vi "live view D04.vi"() -> ()   [LabVIEW 2019, in "D04.lvlib"]
uses:
  D04.lvlib
  <vilib>/userDefined/High Color/IMAQdx.ctl
  <vilib>/vision/Image Controls.llb/IMAQ Image.ctl
  <vilib>/measure/mamon.llb/Trigger Detection for 1 Channel.vi
  <vilib>/measure/NI_MAPro.lvlib
  Calibration Lib.lvlib
  database.lvlib
  <vilib>/vision/driver/NI_Vision_Acquisition_Software.lvlib
panel:
  out "Error out":errorcluster
  in  "Save Button":bool
  in  "Calib IMQ Num":u16(ring) items=["First IMQ", "Second IMQ", "Third IMQ"]
  in  "Verify Calibration1 D04":bool caption="capture grab"
  in  "snapshot":bool
  out "error prj03":errorcluster
  in  "Verify Calibration D04":bool caption="capture grab"
  in  "Close":bool
  in  "Method 2 save D04":bool caption="capture grab"
  in  "Method 1 Save D04":bool caption="Saving txt"
  out "Average Result":string="Average Result"
  out ">18  A":dbl(slide)=1.0 caption=">16 mm" scale=0.0..100.0
  out "16-18  A":dbl(slide)=1.0 caption="14-16 mm" scale=0.0..100.0
  out "14-16  A":dbl(slide)=1.0 caption="12.7-14 mm" scale=0.0..100.0
  out "12.5-14 A":dbl(slide)=1.0 caption="11-12.7 mm" scale=0.0..100.0
  out "10-12.5  A":dbl(slide)=1.0 caption="9.5-11 mm" scale=0.0..100.0 scale format="%#_4f"
  out "8-10  A":dbl(slide)=1.0 caption="8-9.5 mm" scale=0.0..100.0
  out "6.3-8  A":dbl(slide)=1.0 caption="6.3-8 mm" scale=0.0..100.0
  out "<6.3  A":dbl(slide)=1.0 caption="<6.3 mm" scale=0.0..100.0
  out "Live Result":string="Live Result"
  out ">18  L":dbl(slide)=1.0 caption=">16 mm" scale=0.0..100.0
  out "Live View":T1(plugin-control) caption="Disc 26"
  out "16-18  L":dbl(slide)=1.0 caption="14-16 mm" scale=0.0..100.0
  out "14-16  L":dbl(slide)=1.0 caption="12.7-14 mm" scale=0.0..100.0
  out "12.5-14 L":dbl(slide)=1.0 caption="11-12.7 mm" scale=0.0..100.0
  out "10-12.5  L":dbl(slide)=1.0 caption="9.5-11 mm" scale=0.0..100.0 scale format="%#_4f"
  out "8-10  L":dbl(slide)=1.0 caption="8-9.5 mm" scale=0.0..100.0
  out "6.3-8  L":dbl(slide)=1.0 caption="6.3-8 mm" scale=0.0..100.0
  out "<6.3  L":dbl(slide)=1.0 caption="<6.3 mm" scale=0.0..100.0
  out "disc name":string="Live Info Disc 04"
  out "dsgs":string="DSGS"
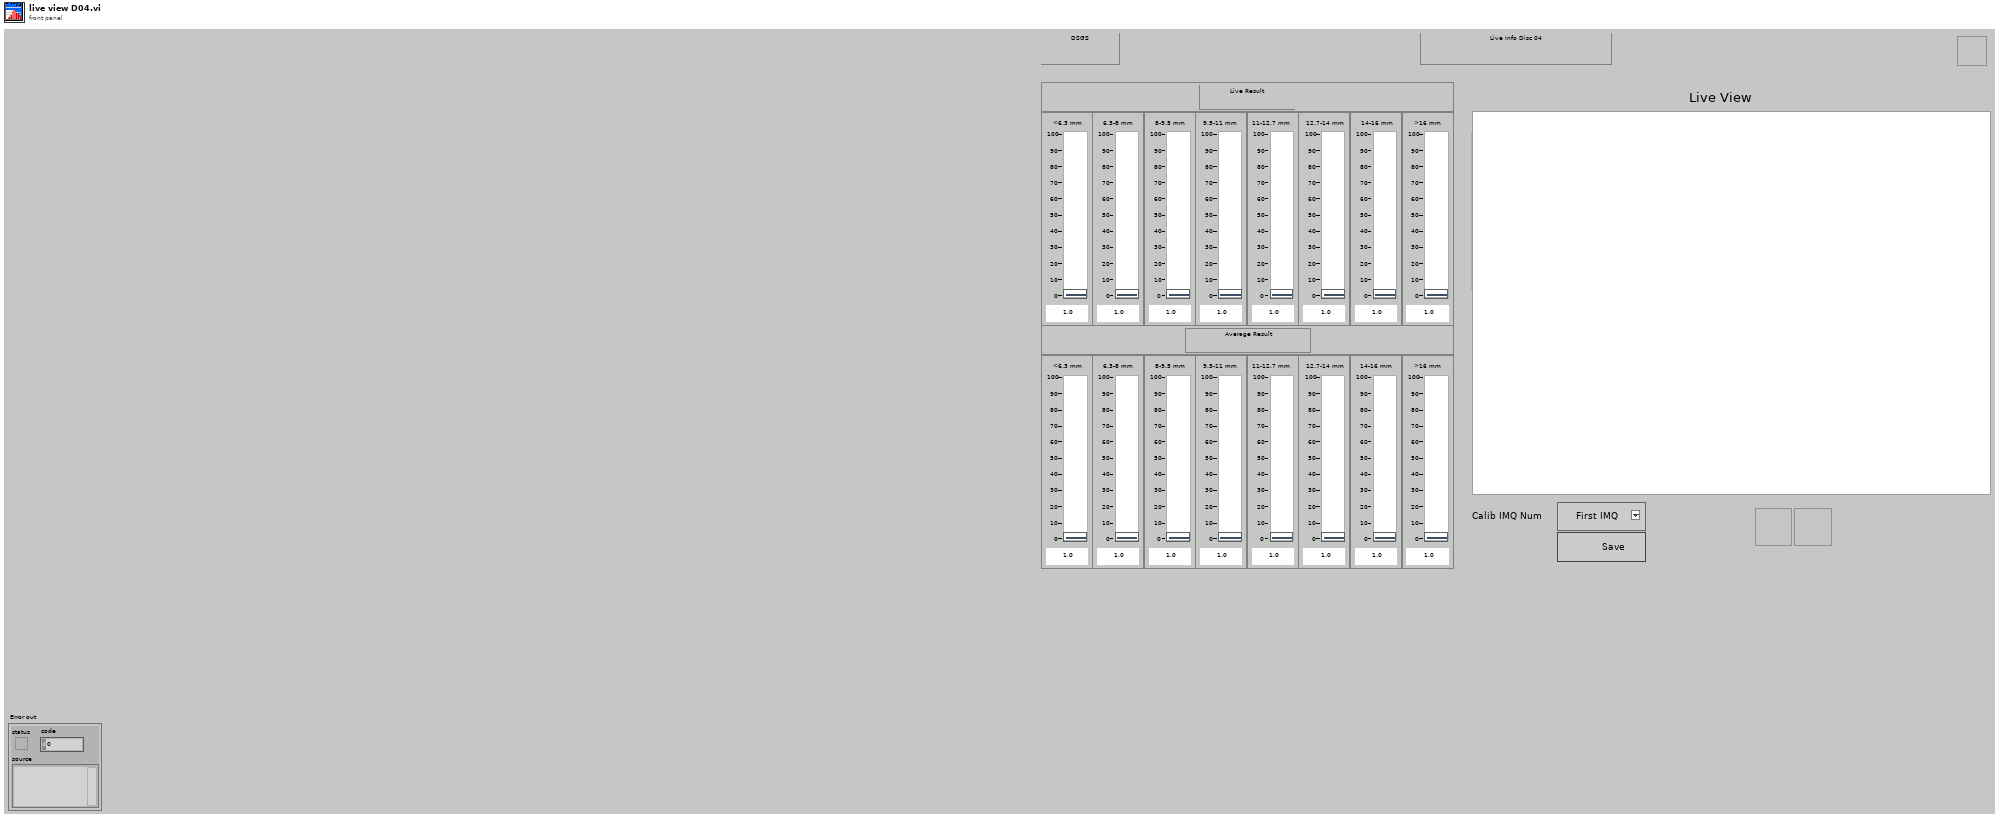
[diagram p1: front panel]
types:
  T1 = typedef "IMAQ Image.ctl" = refnum<image>
  T2 = typedef "IMAQdx.ctl" = refnum<k21>
  T3 = enum8{"Enabled", "Disabled", "Disabled and Grayed Out"}
  T4 = cluster{"date/time string":string, "date/time string":string, string, "Value":dbl, "Value":dbl, "Value":dbl, "Value":dbl, "Value":dbl, "Value":dbl, "Value":dbl, "Value":dbl}
  T5 = cluster{"date/time string":string, "date/time string":string, i32, "spreadsheet string":string, "spreadsheet string":string}
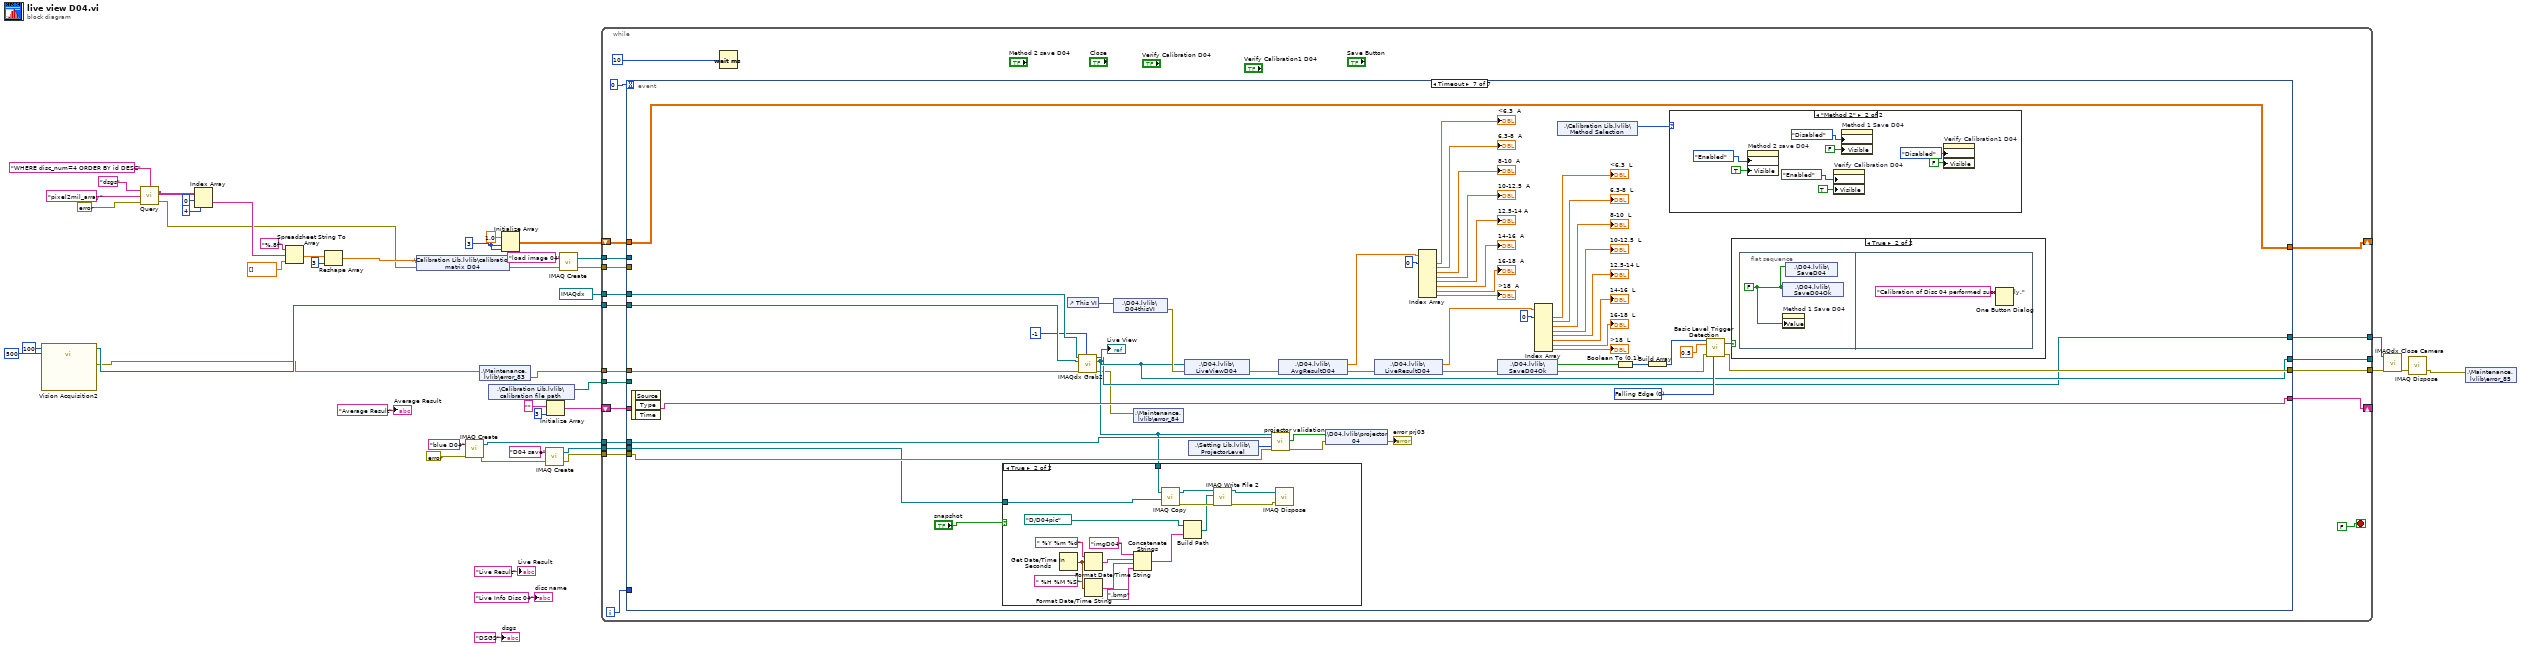
[diagram p0: block diagram]
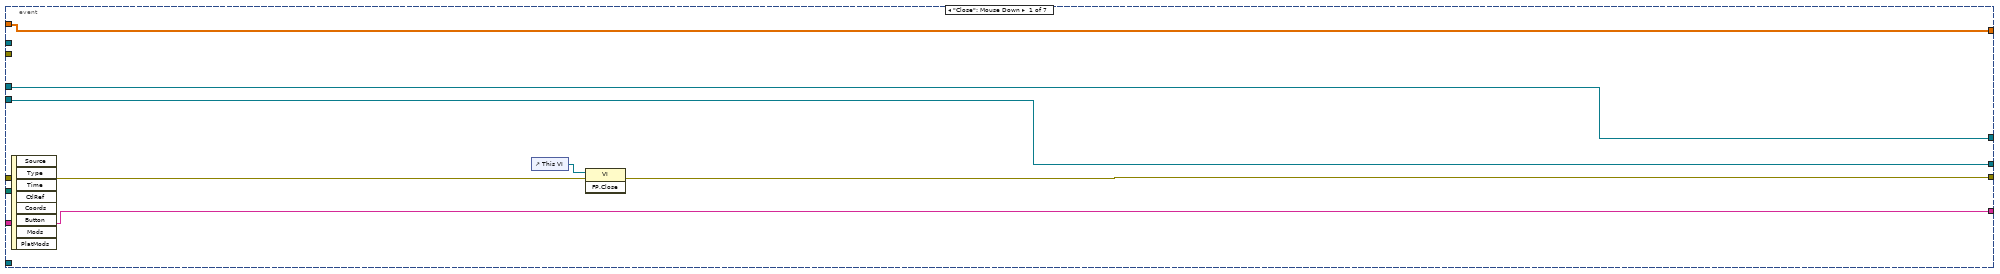
[diagram p2: hidden frame]
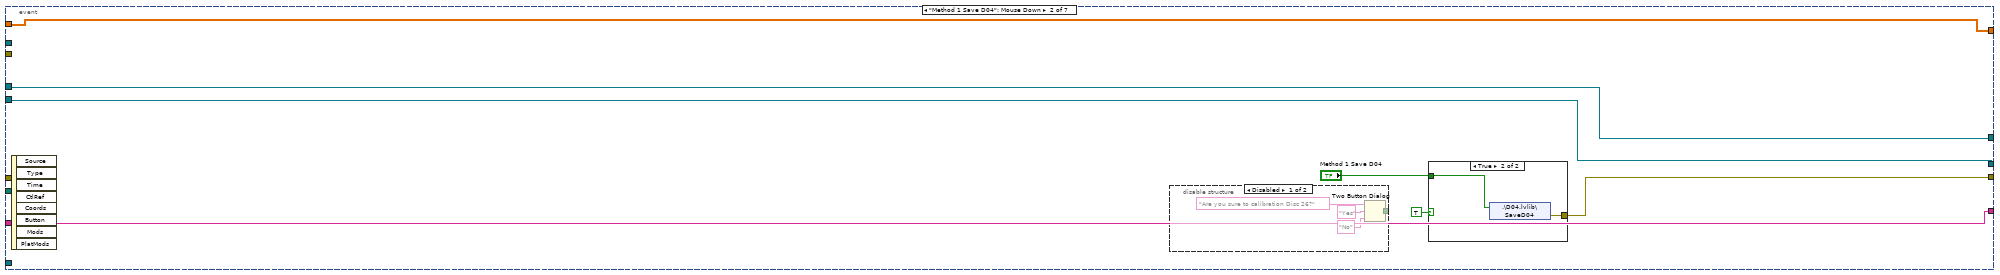
[diagram p3: hidden frame]
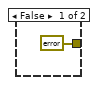
[diagram p5: hidden frame]
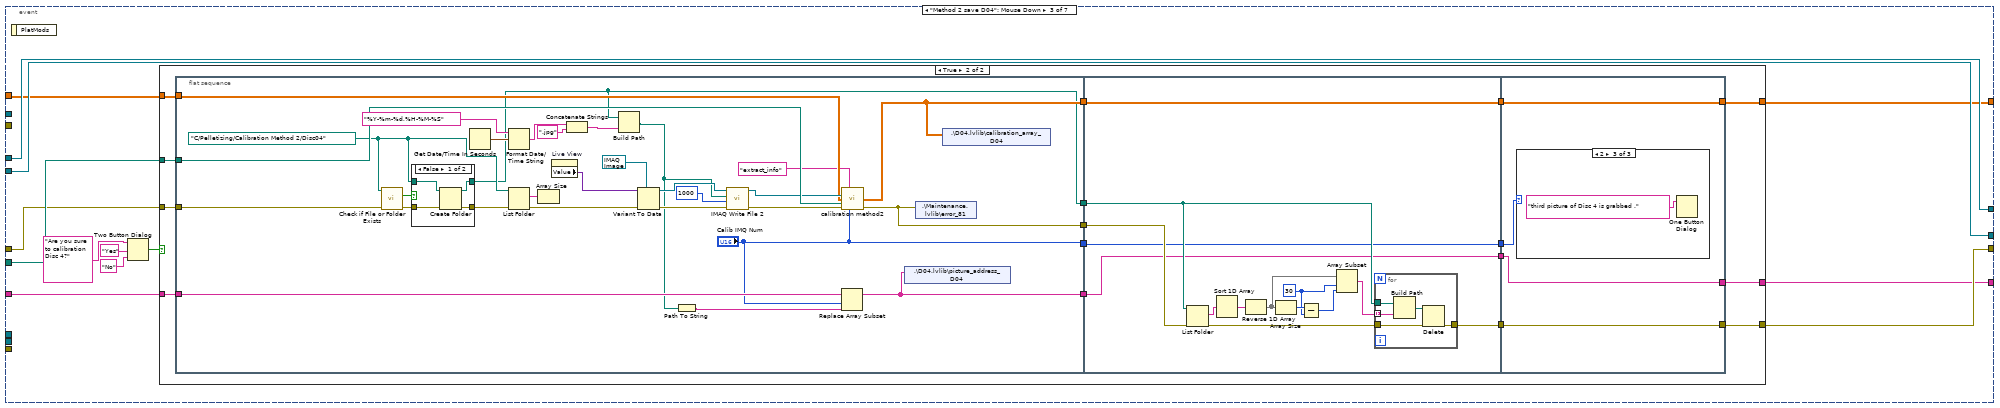
[diagram p6: hidden frame]
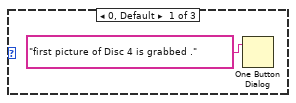
[diagram p9: hidden frame]
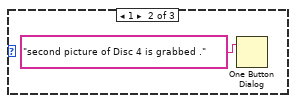
[diagram p10: hidden frame]
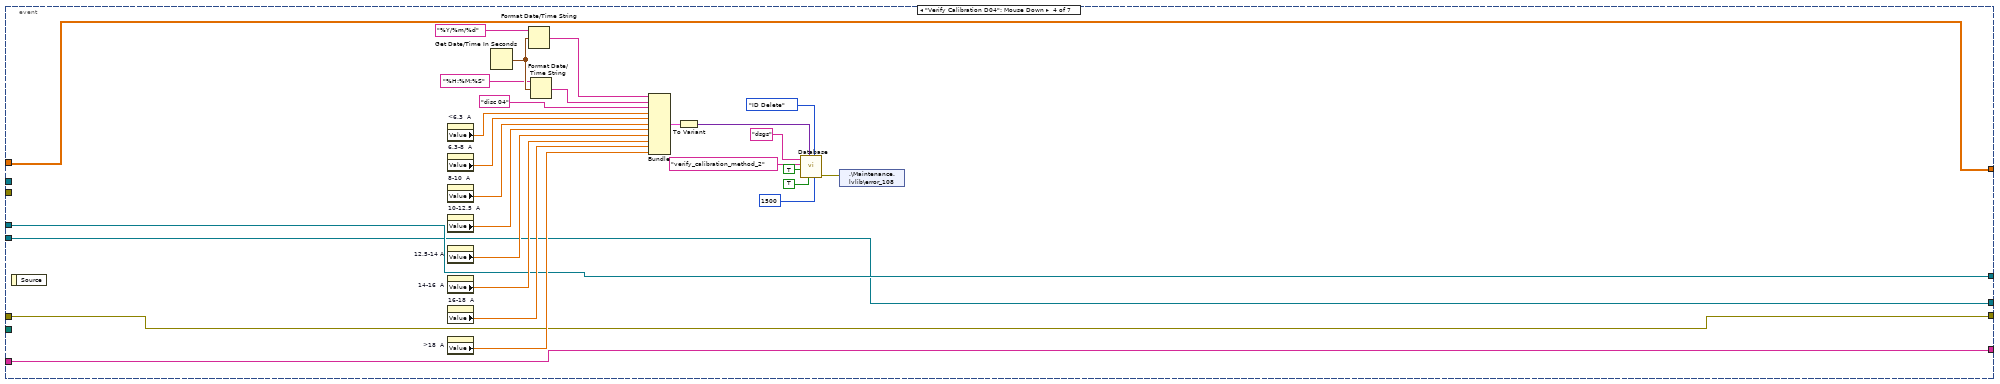
[diagram p11: hidden frame]
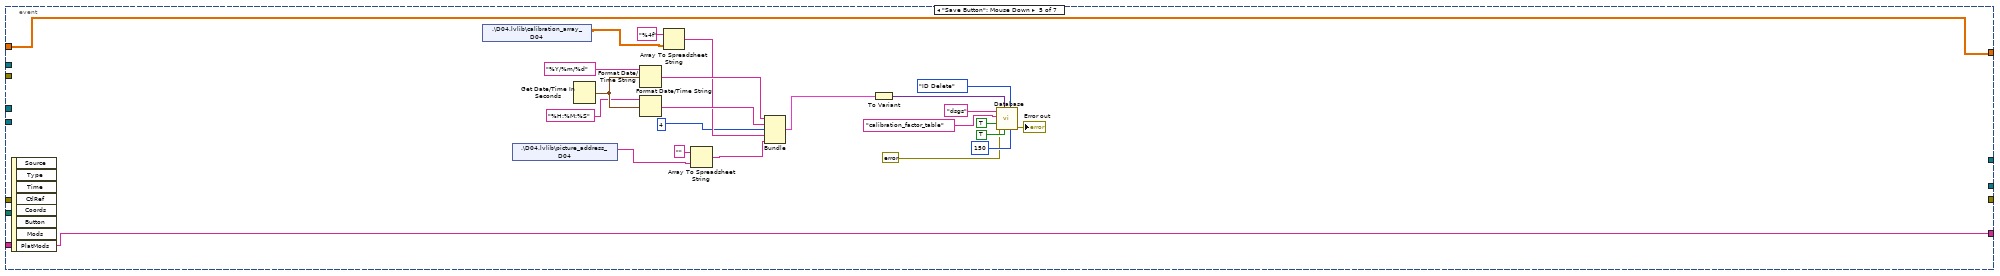
[diagram p12: hidden frame]
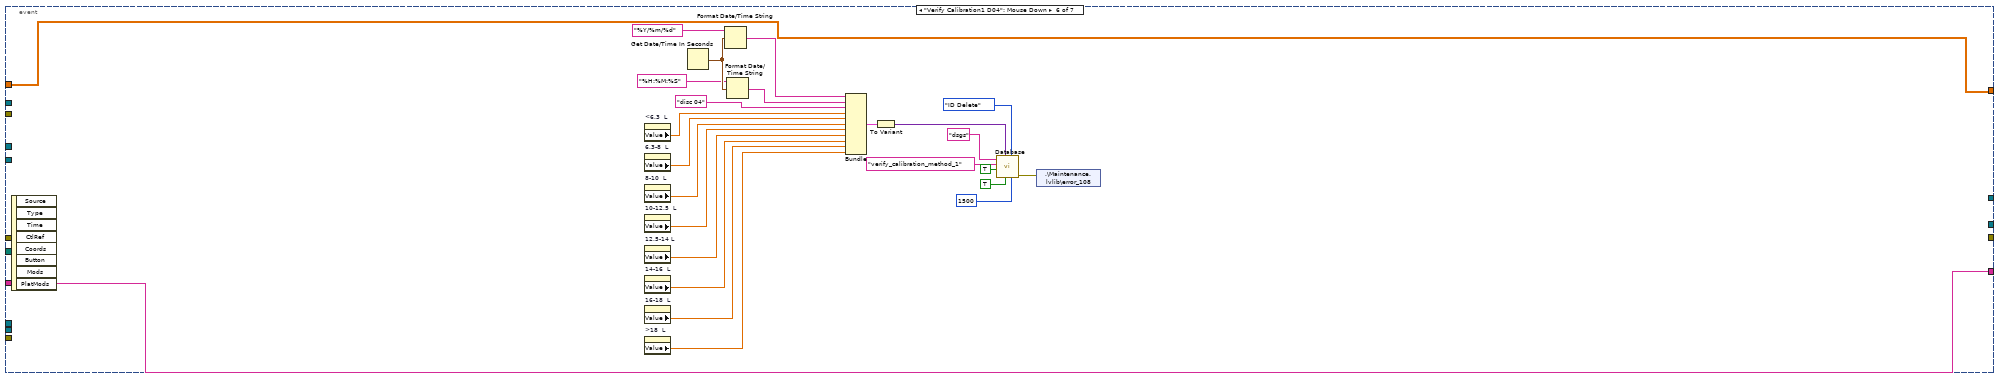
[diagram p13: hidden frame]
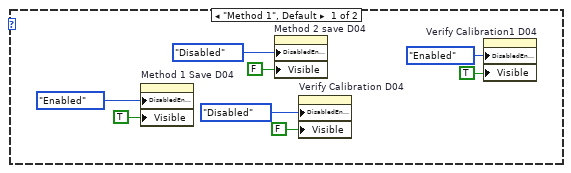
[diagram p15: hidden frame]
diagram:
  w15 = 3 ("dimension size")
  n1 = call "Vision Acquisition2"("Gain (Raw)"=i64 100, "Exposure Time (Raw)"=i64 500) -> ("Image Out"=w4:T1, "error out"=w3:errorcluster)  [unwired: 23 in, 1 out]
  n2 = call "Query.vi"("Condition"="WHERE disc_num=4 ORDER BY id DESC", "Error in"=errorcluster {"status"=FALSE, "code"=0, "source"=""}, "Table Name"="pixel2mil_array", "Connection Name"="dsgs") -> ("Error out"=w7:errorcluster, "data"=w10:string[][])
  n3 = Index Array(array=w10, index (row)=0, index (col)=4 ("disabled index (col)")) -> (element=w8:string)
  n4 = Spreadsheet String To Array(format string="%.8f", spreadsheet string=w8, array type (2D Dbl)=sgl[] []) -> (array=w28:sgl[])  [unwired: 1 in]
  n5 = Reshape Array(w28, 3 ("dimension size")) -> (w25:sgl[])
  n6 = shared-variable ".\\Calibration Lib.lvlib\\calibration matrix D04"(w25, error in=w7) -> (error out=w24:errorcluster)
  n7 = call "IMAQ Create"("Image Name"="blue D04", "error in (no error)"=errorcluster {"status"=FALSE, "code"=0, "source"=""}) -> ("New Image"=w22:T1, "error out"=w20:errorcluster)  [unwired: 3 in]
  n8 = shared-variable ".\\Maintenance.lvlib\\error_83"(w3) -> (error out=w37:errorcluster)  [unwired: 1 in]
  n9 = shared-variable ".\\Calibration Lib.lvlib\\calibration file path"() -> (w38:path)  [unwired: 1 in, 1 out]
  n10 = Initialize Array(1.0 ("element"), w15, w15) -> (w14:dbl[][])
  n11 = call "IMAQ Create"("Image Name"="D04 save", "error in (no error)"=w20) -> ("New Image"=w17:T1, "error out"=w19:errorcluster)  [unwired: 3 in]
  n12 = Initialize Array("", 3 ("dimension size")) -> (w11:string[])
  n13 = call "IMAQ Create"("Image Name"="load image 04", "error in (no error)"=w24) -> ("New Image"=w34:T1, "error out"=w35:errorcluster)  [unwired: 3 in]
  n14 = while {
    tunnel: w38 -> [w64]
    tunnel: w37 -> [w63]
    tunnel: w4 -> [w61]
    tunnel: [w60] -> w42
    tunnel: [w59] -> _
    tunnel: T2 "cam3" ("Session In") -> [w58]
    tunnel: [w57] -> w39
    tunnel: w35 -> [w56]
    tunnel: w34 -> [w55]
    tunnel: w22 -> [w54]
    tunnel: w19 -> [w53]
    tunnel: w17 -> [w52]
    shift-right: [w49] -> _
    shift-left: w14 -> [w50]
    shift-right: [w47] -> _
    shift-left: w11 -> [w48]
    i -> [w51]
    stop <- FALSE stop-if-true
    n15 = event shown="[6] Timeout" {
      selector: _ -> [_ _ _ _ _ _ _]
      dyn-events: _ -> [_ _ _ _ _ _ _]
      timeout: 0 -> [_ _ _ _ _ _ _]
      tunnel: w64 -> [_ _ w100 _ _ _ _]
      tunnel: [w72 w80 w96 w188 _ _ w277] -> w60
      tunnel: w63 -> [w71 _ w99 w188 _ _ w262]
      tunnel: w61 -> [w70 w79 w98 w186 _ _ w261]
      tunnel: [w70 w79 w98 w186 _ _ w265] -> w59
      tunnel: w58 -> [w69 w78 w97 w187 _ _ w264]
      tunnel: [w69 w78 w97 w187 _ _ w263] -> w57
      tunnel: w56 -> [_ _ _ _ _ _ _]
      tunnel: w55 -> [_ _ _ _ _ _ _]
      tunnel: w54 -> [_ _ _ _ _ _ w275]
      tunnel: w53 -> [_ _ _ _ _ _ w271]
      tunnel: w52 -> [_ _ _ _ _ _ w268]
      tunnel: w51 -> [_ _ _ _ _ _ _]
      tunnel: w50 -> [w68 w75 w91 w183 w212 w235 w267]
      tunnel: [w68 w75 w90 w183 w212 w235 w267] -> w49
      tunnel: w48 -> [w67 w74 w89 w182 w211 w234 w266]
      tunnel: [w67 w74 w88 w182 w211 w234 w266] -> w47
      event "Close": Mouse Down {
        n16 = event-data() -> ()  [unwired: 1 in, 8 out]
        n17 = control-ref of="This VI"() -> (w73:refnum<vi>)
        n18 = invoke class="VI" method="FP.Close"(reference=w73, error in=w71) -> (error out=w72:errorcluster)  [unwired: 1 in, 2 out]
      }
      event "Method 1 Save D04": Mouse Down {
        n19 = event-data() -> ()  [unwired: 1 in, 8 out]
        n20 = disable-structure shown="Disabled" {
          disable-tunnel: [w81 _] -> _
          frame Disabled {
            n21 = Two Button Dialog(message="Are you sure to calibration Disc 26?", 1:"No" ("F button name (\"Cancel\")"), 2:"Yes" ("T button name (\"OK\")")) -> (T button?=w81:bool)
          }
          frame Enabled {
          }
        }
        n22 = case shown="True" TRUE {
          tunnel: [errorcluster {"status"=FALSE, "code"=0, "source"=""} ("error IO") w87] -> w80
          tunnel: "Method 1 Save D04" -> [_ w86]
          frame False {
          }
          frame True {
            n23 = shared-variable ".\\D04.lvlib\\SaveD04"(w86) -> (error out=w87:errorcluster)  [unwired: 1 in]
          }
        }
      }
      event "Method 2 save D04": Mouse Down {
        n24 = event-data() -> ()  [unwired: 1 in, 1 out]
        n25 = Two Button Dialog(message="Are you sure to calibration Disc 4?", 1:"No" ("F button name (\"Cancel\")"), 2:"Yes" ("T button name (\"OK\")")) -> (T button?=w92:bool)
        n26 = case shown="True" w92 {
          tunnel: w100 -> [_ w118]
          tunnel: w99 -> [w103 w117]
          tunnel: [w103 w116] -> w96
          tunnel: w91 -> [w102 w114]
          tunnel: [w102 w111] -> w90
          tunnel: w89 -> [w101 w110]
          tunnel: [w101 w107] -> w88
          frame False {
          }
          frame True {
            n27 = flat-sequence {
              tunnel: w117 -> [w138]
              tunnel: w118 -> [w149]
              tunnel: [w123] -> w119
              tunnel: w114 -> [w131]
              tunnel: [w130] -> w112
              tunnel: w110 -> [w127]
              tunnel: [w126] -> w108
              tunnel: [w125] -> w106
              tunnel: ["Calib IMQ Num"] -> w104
              tunnel: [w160] -> w115
              tunnel: [w158] -> w113
              tunnel: [w157] -> w109
              tunnel: w106 -> [w161]
              tunnel: w108 -> [w157]
              tunnel: w112 -> [w158]
              tunnel: w119 -> [w162]
              tunnel: [w156] -> w105
              tunnel: w104 -> [w156]
              tunnel: [w178] -> w116
              tunnel: w115 -> [w178]
              tunnel: [w177] -> w111
              tunnel: w113 -> [w177]
              tunnel: [w176] -> w107
              tunnel: w109 -> [w176]
              tunnel: w105 -> [w175]
              frame #0 {
                w134 = path "C:/Pelletizing/Calibration Method 2/Disc04" ("path")
                n28 = call <vilib>:"Check if File or Folder Exists.vi"("error in (no error)"=w138, "path"=w134) -> ("error out"=w139:errorcluster, "file or folder exists?"=w140:bool)  [unwired: 7 in, 1 out]
                n29 = case shown="False" w140 {
                  tunnel: [w151 w155] -> w123
                  tunnel: w134 -> [w153 w155]
                  tunnel: w139 -> [w152 w154]
                  tunnel: [w150 w154] -> w136
                  frame False {
                    n30 = Create Folder(path (use dialog)=w153, error in=w152) -> (created path=w151:path, error out=w150:errorcluster)  [unwired: 1 in, 1 out]
                  }
                  frame True {
                  }
                }
                n31 = Get Date/Time In Seconds() -> (seconds since 1Jan1904=w144:timestamp)
                n32 = Format Date/Time String(time format string (%c)="%Y-%m-%d,%H-%M-%S", seconds (now)=w144) -> (date/time string=w142:string)  [unwired: 1 in]
                n33 = List Folder(path=w134, error in=w136) -> (filenames=w137:string[], error out=w135:errorcluster)  [unwired: 2 in, 2 out]
                n34 = Array Size(array=w137) -> ()  [unwired: 1 out]
                n35 = property on="Live View" class="ImageControl"() -> ("Value"=w148:variant)  [unwired: 2 in, 2 out]
                n36 = Concatenate Strings(w142, ".jpg" ("string")) -> (w124:string)
                n37 = Build Path(base path=w123, name or relative path=w124) -> (appended path=w121:path)
                n38 = Variant To Data(error in=w135, type=T1 refnum ("New Image"), Variant=w148) -> (data=w132:T1, error out=w145:errorcluster)
                n39 = Path To String(path=w121) -> (string=w122:string)
                n40 = call-poly "IMAQ Write File 2"("error in (no error)"=w145, "Image Quality"=u32 1000, "File Path"=w121, "Image"=w132) -> ("error out"=w129:errorcluster, "Image Out (duplicate)"=w133:T1)  [unwired: 6 in]
                n41 = Replace Array Subset(array=w127, new element=w122, index="Calib IMQ Num") -> (w126:string[])
                n42 = call "calibration method2.vi"("function name"="extract_info", "Image IN"=w133, "initialize matrix"=w131, "module path"=w149, "error in"=w129, "snap number"="Calib IMQ Num") -> ("calibration matrix"=w130:dbl[][], "error out"=w125:errorcluster)  [unwired: 8 in]
                n43 = shared-variable ".\\D04.lvlib\\picture_address_D04"(w126) -> ()  [unwired: 1 in, 1 out]
                n44 = shared-variable ".\\Maintenance.lvlib\\error_81"(w125) -> ()  [unwired: 1 in, 1 out]
                n45 = shared-variable ".\\D04.lvlib\\calibration_array_D04"(w130) -> ()  [unwired: 1 in, 1 out]
              }
              frame #1 {
                w163 = 30 ("index")
                n46 = List Folder(path=w162, error in=w161) -> (filenames=w169:string[], error out=w159:errorcluster)  [unwired: 2 in, 2 out]
                n47 = Sort 1D Array(array=w169) -> (sorted array=w168:string[])
                n48 = Reverse 1D Array(array=w168) -> (reversed array=w167:string[])
                n49 = Array Size(array=w167) -> (size(s)=w166:i32)
                n50 = Subtract(x=w166, y=w163) -> (x-y=w165:i32)
                n51 = Array Subset(array=w167, index=w163, length=w165) -> (w164:string[])
                n52 = for {
                  tunnel: w164 -> [w173] mode=indexing
                  tunnel: w162 -> [w174]
                  tunnel: [w171] -> w160
                  tunnel: w159 -> [w170]
                  n53 = Build Path(base path=w174, name or relative path=w173) -> (appended path=w172:path)
                  n54 = Delete(path (use dialog)=w172, error in=w170) -> (error out=w171:errorcluster)  [unwired: 3 in, 2 out]
                }
              }
              frame #2 {
                n55 = case shown="2" w175 {
                  frame 0, Default {
                    n56 = One Button Dialog(message="first picture of Disc 4 is grabbed .") -> ()  [unwired: 1 in, 1 out]
                  }
                  frame 1 {
                    n57 = One Button Dialog(message="second picture of Disc 4 is grabbed .") -> ()  [unwired: 1 in, 1 out]
                  }
                  frame 2 {
                    n58 = One Button Dialog(message="third picture of Disc 4 is grabbed .") -> ()  [unwired: 1 in, 1 out]
                  }
                }
              }
            }
          }
        }
      }
      event "Verify Calibration D04": Mouse Down {
        n59 = event-data() -> ()  [unwired: 1 in, 1 out]
        n60 = property on="<6.3  A" class="Slide (strict)"() -> ("Value"=w203:dbl)  [unwired: 2 in, 2 out]
        n61 = property on="6.3-8  A" class="Slide (strict)"() -> ("Value"=w202:dbl)  [unwired: 2 in, 2 out]
        n62 = property on="8-10  A" class="Slide (strict)"() -> ("Value"=w201:dbl)  [unwired: 2 in, 2 out]
        n63 = property on="10-12.5  A" class="Slide (strict)"() -> ("Value"=w200:dbl)  [unwired: 2 in, 2 out]
        n64 = property on="12.5-14 A" class="Slide (strict)"() -> ("Value"=w199:dbl)  [unwired: 2 in, 2 out]
        n65 = property on="14-16  A" class="Slide (strict)"() -> ("Value"=w198:dbl)  [unwired: 2 in, 2 out]
        n66 = property on="16-18  A" class="Slide (strict)"() -> ("Value"=w197:dbl)  [unwired: 2 in, 2 out]
        n67 = property on=">18  A" class="Slide (strict)"() -> ("Value"=w196:dbl)  [unwired: 2 in, 2 out]
        n68 = Get Date/Time In Seconds() -> (seconds since 1Jan1904=w208:timestamp)
        n69 = Format Date/Time String(time format string (%c)="%Y/%m/%d", seconds (now)=w208) -> (date/time string=w206:string)  [unwired: 1 in]
        n70 = Format Date/Time String(time format string (%c)="%H:%M:%S", seconds (now)=w208) -> (date/time string=w205:string)  [unwired: 1 in]
        n71 = Bundle("date/time string"=w206, "date/time string"=w205, "disc 04", "Value"=w203, "Value"=w202, "Value"=w201, "Value"=w200, "Value"=w199, "Value"=w198, "Value"=w197, "Value"=w196) -> (w195:T4)  [unwired: 1 in]
        n72 = To Variant(anything=w195) -> (Variant=w194:variant)
        n73 = call "Database.vi"("Maximum Row"=1500, "Enum"=enum16{"ID Delete", "Time Delete"}."ID Delete", "Delete row?"=TRUE, "Data"=w194, "Auto Increment ID?"=TRUE, "Table"="verify_calibration_method_2", "Connection"="dsgs") -> ("Error out"=w189:errorcluster)  [unwired: 4 in]
        n74 = shared-variable ".\\Maintenance.lvlib\\error_108"(w189) -> ()  [unwired: 1 in, 1 out]
      }
      event "Save Button": Mouse Down {
        n75 = event-data() -> ()  [unwired: 1 in, 8 out]
        n76 = shared-variable ".\\D04.lvlib\\calibration_array_D04"() -> (w213:dbl[][])  [unwired: 1 in, 1 out]
        n77 = shared-variable ".\\D04.lvlib\\picture_address_D04"() -> (w215:string[])  [unwired: 1 in, 1 out]
        n78 = Get Date/Time In Seconds() -> (seconds since 1Jan1904=w222:timestamp)
        n79 = Format Date/Time String(time format string (%c)="%Y/%m/%d", seconds (now)=w222) -> (date/time string=w223:string)  [unwired: 1 in]
        n80 = Format Date/Time String(time format string (%c)="%H:%M:%S", seconds (now)=w222) -> (date/time string=w221:string)  [unwired: 1 in]
        n81 = Array To Spreadsheet String(array=w213, 3:"%4f" ("format string")) -> (spreadsheet string=w217:string)  [unwired: 1 in]
        n82 = Array To Spreadsheet String(array=w215, 3:"" ("format string")) -> (spreadsheet string=w214:string)  [unwired: 1 in]
        n83 = Bundle("date/time string"=w223, "date/time string"=w221, 4, "spreadsheet string"=w217, "spreadsheet string"=w214) -> (w226:T5)  [unwired: 1 in]
        n84 = To Variant(anything=w226) -> (Variant=w233:variant)
        n85 = call "Database.vi"("Maximum Row"=150, "Enum"=enum16{"ID Delete", "Time Delete"}."ID Delete", "Delete row?"=TRUE, "Data"=w233, "Error in"=errorcluster {"status"=FALSE, "code"=0, "source"=""}, "Auto Increment ID?"=TRUE, "Table"="calibration_factor_table", "Connection"="dsgs") -> ("Error out"=→"Error out":errorcluster)  [unwired: 3 in]
      }
      event "Verify Calibration1 D04": Mouse Down {
        n86 = event-data() -> ()  [unwired: 1 in, 8 out]
        n87 = property on="<6.3  L" class="Slide (strict)"() -> ("Value"=w252:dbl)  [unwired: 2 in, 2 out]
        n88 = property on="6.3-8  L" class="Slide (strict)"() -> ("Value"=w251:dbl)  [unwired: 2 in, 2 out]
        n89 = property on="8-10  L" class="Slide (strict)"() -> ("Value"=w250:dbl)  [unwired: 2 in, 2 out]
        n90 = property on="10-12.5  L" class="Slide (strict)"() -> ("Value"=w249:dbl)  [unwired: 2 in, 2 out]
        n91 = property on="12.5-14 L" class="Slide (strict)"() -> ("Value"=w248:dbl)  [unwired: 2 in, 2 out]
        n92 = property on="14-16  L" class="Slide (strict)"() -> ("Value"=w247:dbl)  [unwired: 2 in, 2 out]
        n93 = property on="16-18  L" class="Slide (strict)"() -> ("Value"=w246:dbl)  [unwired: 2 in, 2 out]
        n94 = property on=">18  L" class="Slide (strict)"() -> ("Value"=w245:dbl)  [unwired: 2 in, 2 out]
        n95 = Get Date/Time In Seconds() -> (seconds since 1Jan1904=w257:timestamp)
        n96 = Format Date/Time String(time format string (%c)="%Y/%m/%d", seconds (now)=w257) -> (date/time string=w255:string)  [unwired: 1 in]
        n97 = Format Date/Time String(time format string (%c)="%H:%M:%S", seconds (now)=w257) -> (date/time string=w254:string)  [unwired: 1 in]
        n98 = Bundle("date/time string"=w255, "date/time string"=w254, "disc 04", "Value"=w252, "Value"=w251, "Value"=w250, "Value"=w249, "Value"=w248, "Value"=w247, "Value"=w246, "Value"=w245) -> (w244:T4)  [unwired: 1 in]
        n99 = To Variant(anything=w244) -> (Variant=w243:variant)
        n100 = call "Database.vi"("Maximum Row"=1500, "Enum"=enum16{"ID Delete", "Time Delete"}."ID Delete", "Delete row?"=TRUE, "Data"=w243, "Auto Increment ID?"=TRUE, "Table"="verify_calibration_method_1", "Connection"="dsgs") -> ("Error out"=w238:errorcluster)  [unwired: 4 in]
        n101 = shared-variable ".\\Maintenance.lvlib\\error_108"(w238) -> ()  [unwired: 1 in, 1 out]
      }
      event Timeout {
        w285 = u16 0 items=["Falling Edge", "Rising Edge"] ("trigger slope")
        n102 = event-data() -> ()  [unwired: 1 in, 3 out]
        n103 = control-ref of="This VI"() -> (w280:refnum<vi>)
        n104 = call <vilib>:"IMAQdx Grab2.vi"("Timeout (ms)"=-1, "error in"=w262, "Image In"=w261, "Session In"=w264) -> ("error out"=w259:errorcluster, "Image Out"=w265:T1, "Session Out"=w263:T2)  [unwired: 4 in, 1 out]
        "Live View" <- w265
        n105 = case shown="True" "snapshot" {
          tunnel: w268 -> [_ w325]
          tunnel: w265 -> [_ w324]
          frame False {
          }
          frame True {
            n106 = Get Date/Time In Seconds() -> (seconds since 1Jan1904=w318:timestamp)
            n107 = Format Date/Time String(time format string (%c)=" %Y %m %d", seconds (now)=w318) -> (date/time string=w314:string)  [unwired: 1 in]
            n108 = Format Date/Time String(time format string (%c)=" %H %M %S", seconds (now)=w318) -> (date/time string=w313:string)  [unwired: 1 in]
            n109 = Concatenate Strings("imgD04" ("string"), w314, w313, ".bmp" ("string")) -> (w311:string)
            n110 = call "IMAQ Copy"("Image Dst"=w325, "Image Src"=w324) -> ("error out"=w322:errorcluster, "Image Dst Out"=w323:T1)  [unwired: 4 in]
            n111 = Build Path(base path=path "D:/D04pic" ("File Path"), name or relative path=w311) -> (appended path=w310:path)
            n112 = call-poly "IMAQ Write File 2"("error in (no error)"=w322, "File Path"=w310, "Image"=w323) -> ("error out"=w320:errorcluster, "Image Out (duplicate)"=w321:T1)  [unwired: 7 in]
            n113 = call "IMAQ Dispose"("Image"=w321, "error in (no error)"=w320) -> ()  [unwired: 4 in, 1 out]
          }
        }
        n114 = shared-variable ".\\D04.lvlib\\D04thisVI"(w280) -> (error out=w276:errorcluster)  [unwired: 1 in]
        n115 = shared-variable ".\\Maintenance.lvlib\\error_84"(w259) -> ()  [unwired: 1 in, 1 out]
        n116 = shared-variable ".\\D04.lvlib\\LiveViewD04"(w265, error in=w276) -> (error out=w279:errorcluster)
        n117 = shared-variable ".\\Setting Lib.lvlib\\ProjectorLevel"() -> (w270:i32)  [unwired: 1 in, 1 out]
        n118 = call "projector validation.vi"("Image Src"=w265, "blue channel"=w275, "on/off level"=w270, "error in (no error)"=w271) -> ("on/off"=w274:bool, "error out"=w273:errorcluster)  [unwired: 14 in]
        n119 = shared-variable ".\\D04.lvlib\\AvgResultD04"(error in=w279) -> (w300:dbl[], error out=w282:errorcluster)
        n120 = shared-variable ".\\D04.lvlib\\projector 04"(w274, error in=w273) -> (error out=→"error prj03":errorcluster)
        n121 = shared-variable ".\\D04.lvlib\\LiveResultD04"(error in=w282) -> (w299:dbl[], error out=w281:errorcluster)
        n122 = Index Array(array=w300, index #1=0 ("index")) -> (element #1=→"<6.3  A":dbl, element #2=→"6.3-8  A":dbl, element #3=→"8-10  A":dbl, element #4=→"10-12.5  A":dbl, element #5=→"12.5-14 A":dbl, element #6=→"14-16  A":dbl, element #7=→"16-18  A":dbl, element #8=→">18  A":dbl)  [unwired: 7 in]
        n123 = shared-variable ".\\D04.lvlib\\SaveD04Ok"(error in=w281) -> (w286:bool, error out=w278:errorcluster)
        n124 = Index Array(array=w299, index #1=0 ("index")) -> (element #1=→"<6.3  L":dbl, element #2=→"6.3-8  L":dbl, element #3=→"8-10  L":dbl, element #4=→"10-12.5  L":dbl, element #5=→"12.5-14 L":dbl, element #6=→"14-16  L":dbl, element #7=→"16-18  L":dbl, element #8=→">18  L":dbl)  [unwired: 7 in]
        n125 = shared-variable ".\\Calibration Lib.lvlib\\Method Selection"() -> (w283:enum32{"Method 1", "Method 2"})  [unwired: 1 in, 1 out]
        n126 = Boolean To (0,1)(Boolean=w286) -> (0, 1=w289:i16)
        n127 = Build Array(w289) -> (w288:i16[])
        n128 = case shown="\"Method 2\"" w283 {
          frame "Method 1", Default {
            n129 = property on="Method 1 Save D04" class="Bool (strict)"("DisabledEnum"=T3."Enabled" ("Disabled"), "Visible"=TRUE) -> ()  [unwired: 2 in, 2 out]
            n130 = property on="Method 2 save D04" class="Bool (strict)"("DisabledEnum"=T3."Disabled" ("Disabled"), "Visible"=FALSE) -> ()  [unwired: 2 in, 2 out]
            n131 = property on="Verify Calibration D04" class="Bool (strict)"("DisabledEnum"=T3."Disabled" ("Disabled"), "Visible"=FALSE) -> ()  [unwired: 2 in, 2 out]
            n132 = property on="Verify Calibration1 D04" class="Bool (strict)"("DisabledEnum"=T3."Enabled" ("Disabled"), "Visible"=TRUE) -> ()  [unwired: 2 in, 2 out]
          }
          frame "Method 2" {
            n133 = property on="Method 2 save D04" class="Bool (strict)"("DisabledEnum"=T3."Enabled" ("Disabled"), "Visible"=TRUE) -> ()  [unwired: 2 in, 2 out]
            n134 = property on="Verify Calibration D04" class="Bool (strict)"("DisabledEnum"=T3."Enabled" ("Disabled"), "Visible"=TRUE) -> ()  [unwired: 2 in, 2 out]
            n135 = property on="Method 1 Save D04" class="Bool (strict)"("DisabledEnum"=T3."Disabled" ("Disabled"), "Visible"=FALSE) -> ()  [unwired: 2 in, 2 out]
            n136 = property on="Verify Calibration1 D04" class="Bool (strict)"("DisabledEnum"=T3."Disabled" ("Disabled"), "Visible"=FALSE) -> ()  [unwired: 2 in, 2 out]
          }
        }
        n137 = call-poly <vilib>:"Basic Level Trigger Detection.vi"("signal in"=w288, "level"=0.5, "error in (no error)"=w278, "trigger slope"=w285) -> ("trigger detected?"=w284:bool, "error out"=w277:errorcluster)  [unwired: 9 in, 1 out]
        n138 = case shown="True" w284 {
          frame False {
          }
          frame True {
            n139 = flat-sequence {
              frame #0 {
                w342 = FALSE
                n140 = shared-variable ".\\D04.lvlib\\SaveD04Ok"(w342) -> ()  [unwired: 1 in, 1 out]
                n141 = property on="Method 1 Save D04" class="Bool (strict)"("Value"=w342) -> ()  [unwired: 2 in, 2 out]
                n142 = shared-variable ".\\D04.lvlib\\SaveD04"(w342) -> ()  [unwired: 1 in, 1 out]
              }
              frame #1 {
                n143 = One Button Dialog(message="Calibration of Disc 04 performed successfully.") -> ()  [unwired: 1 in, 1 out]
              }
            }
          }
        }
      }
    }
    n144 = Wait (ms)(milliseconds to wait=u32 10) -> ()  [unwired: 1 out]
  }
  n145 = call <vilib>:"IMAQdx Close Camera.vi"("error in"=w42, "Session In"=w39) -> ("error out"=w41:errorcluster)  [unwired: 9 in]
  n146 = call "IMAQ Dispose"("error in (no error)"=w41) -> ("error out"=w5:errorcluster)  [unwired: 5 in]
  n147 = shared-variable ".\\Maintenance.lvlib\\error_85"(w5) -> ()  [unwired: 1 in, 1 out]
  "Live Result" <- "Live Result" ("Live Result")
  "Average Result" <- "Average Result" ("Average Result")
  "disc name" <- "Live Info Disc 04" ("Live Result")
  "dsgs" <- "DSGS" ("Live Result")
